vi "PositionTest.vi"() -> ()   [LabVIEW 2011]
uses:
  <vilib>/Analysis/NI_AALBase.lvlib
panel:
  out "OverTravelReached":bool
  in  "Minimum Position":dbl=10000.0
  out "MaxError":dbl[](array[numeric])
  out "MinError":dbl[](array[numeric])
  out "Positive Error":T1(graph)={"X Values"=[50.6, 51.8, 53.0, 54.2, 55.4, 56.6, 57.8, 59.0, 60.2, 61.4], "Histogram: h(x)"=[4, 6, 12, 22, 11, 20, 13, 12, 8, 2]}
  out "Negative Error":T1(graph)={"X Values"=[50.6, 51.8, 53.0, 54.2, 55.4, 56.6, 57.8, 59.0, 60.2, 61.4], "Histogram: h(x)"=[4, 6, 12, 22, 11, 20, 13, 12, 8, 2]}
  out "VRN":refnum<visa-resource-name>="COM10"
  in  "STOP":bool
  in  "GO":bool
  in  "Maximum Position":dbl=10000.0
  in  "Accel_A":dbl=20000.0
  in  "Fast_A":dbl=30000.0
  in  "Slow_A":dbl=1.0
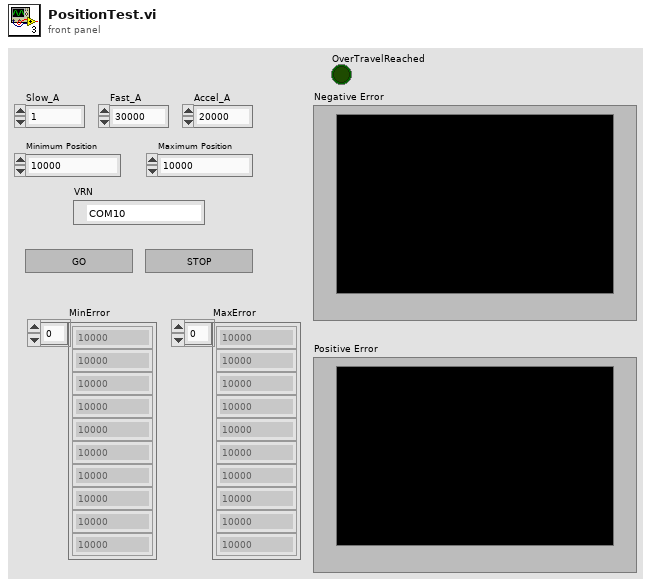
[diagram p1: front panel]
types:
  T1 = cluster{"X Values":dbl[], "Histogram: h(x)":i32[]}
  T2 = enum8{"Enabled", "Disabled", "Disabled and Grayed Out"}
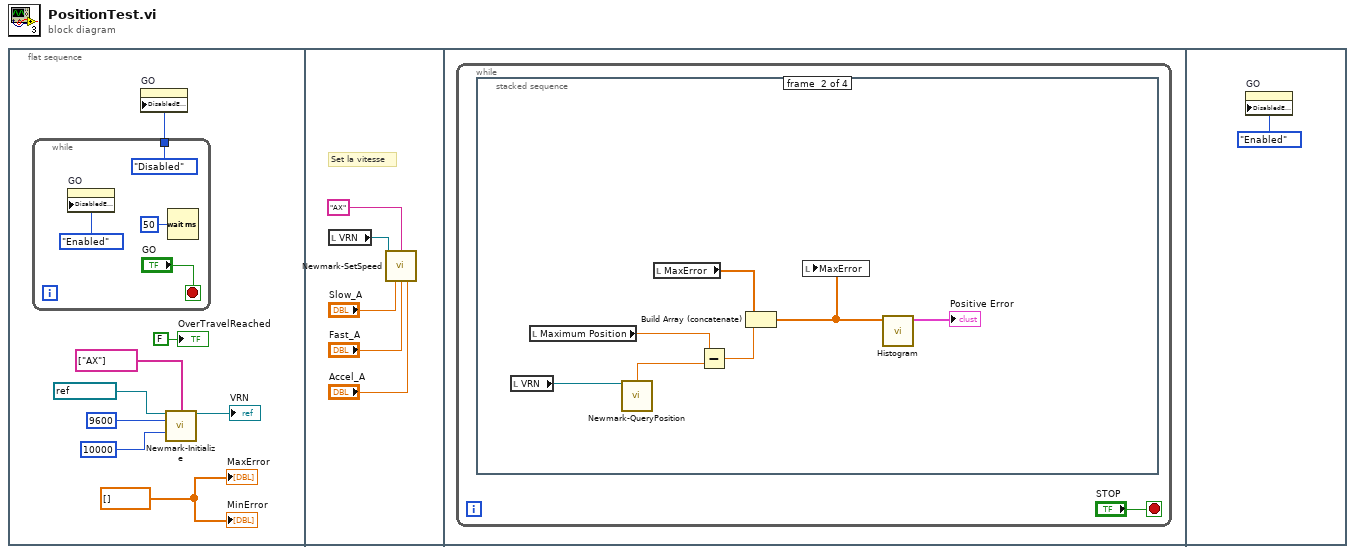
[diagram p0: block diagram]
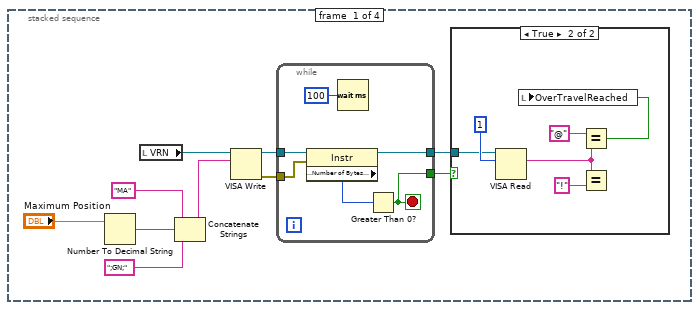
[diagram p2: hidden frame]
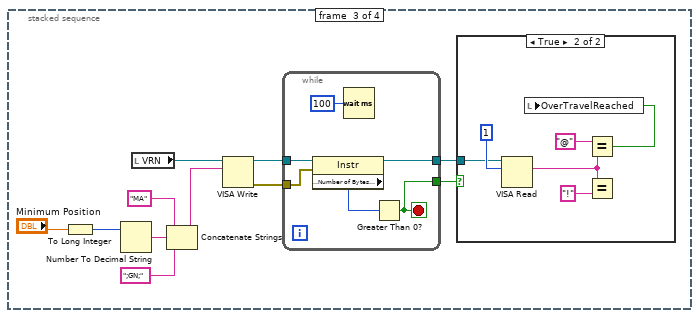
[diagram p4: hidden frame]
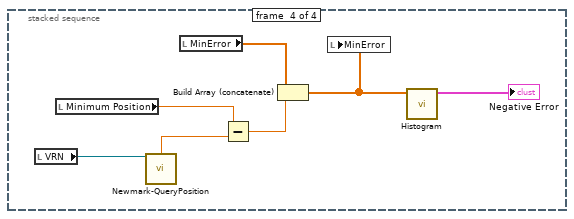
[diagram p6: hidden frame]
diagram:
  n1 = flat-sequence {
    frame #0 {
      w2 = dbl[] [] ("Array")
      n2 = while {
        tunnel: [T2."Disabled" ("Disabled")] -> w8
        stop <- "GO" stop-if-true
        n3 = property on="GO" class="Bool"("DisabledEnum"=T2."Enabled" ("Disabled")) -> ()  [unwired: 2 in, 2 out]
        n4 = Wait (ms)(milliseconds to wait=u32 50) -> ()  [unwired: 1 out]
      }
      n5 = property on="GO" class="Bool"("DisabledEnum"=w8) -> ()  [unwired: 2 in, 2 out]
      n6 = call "Newmark-Initialize.vi"("VISA resource name"=refnum<visa-resource-name> "COM10", "ActiveStages"=string[] ["AX"], "baud rate"=u32 9600, "Timeout"=u32 10000) -> ("VISA resource name out"=→"VRN":refnum<visa-resource-name>)  [unwired: 10 in, 1 out]
      "MaxError" <- w2
      "MinError" <- w2
      "OverTravelReached" <- FALSE ("OverTravelReached")
    }
    frame #1 {
      # "Set la vitesse"
      n7 = local read "VRN"() -> (w16:refnum<visa-resource-name>)
      n8 = call "Newmark-SetSpeed.vi"("Table VRN"=w16, "StageTAG"="AX", "Vitesse Lente"="Slow_A", "Vitesse Rapide"="Fast_A", "Accélération"="Accel_A") -> ()  [unwired: 8 in, 3 out]
    }
    frame #2 {
      n9 = while {
        stop <- "STOP" stop-if-true
        n10 = stacked-sequence {
          frame #0 {
            n11 = Number To Decimal String(number="Maximum Position") -> (decimal integer string=w22:string)  [unwired: 1 in]
            n12 = local read "VRN"() -> (w26:refnum<visa-resource-name>)
            n13 = Concatenate Strings("MA", w22, ";GN;") -> (w21:string)
            n14 = VISA Write(VISA resource name=w26, write buffer=w21) -> (VISA resource name out=w27:refnum<visa-resource-name>, error out=w28:errorcluster)  [unwired: 1 in, 1 out]
            n15 = while {
              tunnel: w27 -> [w39]
              tunnel: w28 -> [w38]
              tunnel: [w36] -> w20
              tunnel: [w35] -> w19
              stop <- w35 stop-if-true
              n16 = property class="Instr"(reference=w39, error in=w38) -> (reference out=w36:refnum<visa-resource-name>, "Serial Settings:Number of Bytes at Serial Port"=w37:u32)  [unwired: 1 out]
              n17 = Wait (ms)(milliseconds to wait=u32 100) -> ()  [unwired: 1 out]
              n18 = Greater Than 0?(x=w37) -> (x > 0?=w35:bool)
            }
            n19 = case shown="True" w19 {
              tunnel: w20 -> [_ w29]
              frame False {
              }
              frame True {
                n20 = VISA Read(VISA resource name=w29, byte count=u32 1) -> (read buffer=w33:string)  [unwired: 1 in, 3 out]
                n21 = Equal?(x="@", y=w33) -> (x = y?=w30:bool)
                n22 = local write "OverTravelReached"(w30) -> ()
                n23 = Equal?(x=w33, y="!") -> ()  [unwired: 1 out]
              }
            }
          }
          frame #1 {
            n24 = local read "VRN"() -> (w47:refnum<visa-resource-name>)
            n25 = local read "Maximum Position"() -> (w46:dbl)
            n26 = call "Newmark-QueryPosition.vi"("Table VRN IN"=w47) -> ("X Axis"=w42:dbl)  [unwired: 7 in, 7 out]
            n27 = local read "MaxError"() -> (w44:dbl[])
            n28 = Subtract(x=w46, y=w42) -> (x-y=w45:dbl)
            n29 = Build Array (concatenate)(w44, w45) -> (w41:dbl[])
            n30 = local write "MaxError"(w41) -> ()
            n31 = call <vilib>:"Histogram.vi"("X"=w41) -> ("Histogram Graph"=→"Positive Error":T1)  [unwired: 7 in, 3 out]
          }
          frame #2 {
            n32 = To Long Integer(number="Minimum Position") -> (32bit integer=w52:i32)
            n33 = Number To Decimal String(number=w52) -> (decimal integer string=w55:string)  [unwired: 1 in]
            n34 = local read "VRN"() -> (w58:refnum<visa-resource-name>)
            n35 = Concatenate Strings("MA", w55, ";GN;") -> (w54:string)
            n36 = VISA Write(VISA resource name=w58, write buffer=w54) -> (VISA resource name out=w49:refnum<visa-resource-name>, error out=w48:errorcluster)  [unwired: 1 in, 1 out]
            n37 = while {
              tunnel: w49 -> [w69]
              tunnel: w48 -> [w68]
              tunnel: [w66] -> w51
              tunnel: [w65] -> w50
              stop <- w65 stop-if-true
              n38 = property class="Instr"(reference=w69, error in=w68) -> (reference out=w66:refnum<visa-resource-name>, "Serial Settings:Number of Bytes at Serial Port"=w67:u32)  [unwired: 1 out]
              n39 = Wait (ms)(milliseconds to wait=u32 100) -> ()  [unwired: 1 out]
              n40 = Greater Than 0?(x=w67) -> (x > 0?=w65:bool)
            }
            n41 = case shown="True" w50 {
              tunnel: w51 -> [_ w59]
              frame False {
              }
              frame True {
                n42 = VISA Read(VISA resource name=w59, byte count=u32 1) -> (read buffer=w63:string)  [unwired: 1 in, 3 out]
                n43 = Equal?(x="@", y=w63) -> (x = y?=w60:bool)
                n44 = local write "OverTravelReached"(w60) -> ()
                n45 = Equal?(x=w63, y="!") -> ()  [unwired: 1 out]
              }
            }
          }
          frame #3 {
            n46 = local read "VRN"() -> (w77:refnum<visa-resource-name>)
            n47 = local read "Minimum Position"() -> (w76:dbl)
            n48 = call "Newmark-QueryPosition.vi"("Table VRN IN"=w77) -> ("X Axis"=w73:dbl)  [unwired: 7 in, 7 out]
            n49 = local read "MinError"() -> (w74:dbl[])
            n50 = Subtract(x=w76, y=w73) -> (x-y=w75:dbl)
            n51 = Build Array (concatenate)(w74, w75) -> (w71:dbl[])
            n52 = local write "MinError"(w71) -> ()
            n53 = call <vilib>:"Histogram.vi"("X"=w71) -> ("Histogram Graph"=→"Negative Error":T1)  [unwired: 7 in, 3 out]
          }
        }
      }
    }
    frame #3 {
      n54 = property on="GO" class="Bool"("DisabledEnum"=T2."Enabled" ("Disabled")) -> ()  [unwired: 2 in, 2 out]
    }
  }
